vi "MotorRefNum_Simulation_Global.vi"(0 "menu":enum16{"set", "get", "delete"}(ring)=enum."get", 7 "PWM Channel":T1=enum."PWM 1", 9 "DC Motor Controller Set":refnum<class "DC Motor Controller.lvclass">, 11 "error in (no error)":errorcluster) -> (10 "DC Motor Controller Get":refnum<class "DC Motor Controller.lvclass">, 15 "error out":errorcluster)   [LabVIEW 2017]
doc: "Sets a reference into a registry, gets a reference from a registry, or deletes a reference from a registry. The reference is accessed by name, and can be given any unique name.\n\nThis software is licensed. Open the labview\\readme\\WPI Robotics Library Open Source License.txt file for more information."
uses:
  <instrlib>/DC Motor Controller/HAIOL/DC Motor Controller.lvclass
  <vilib>/Rock Robotics/SystemInterfaces/DIO/FPGA_DIOPWMChannel.ctl
panel:
  out "Array":refnum<class "DC Motor Controller.lvclass">[](array[class])
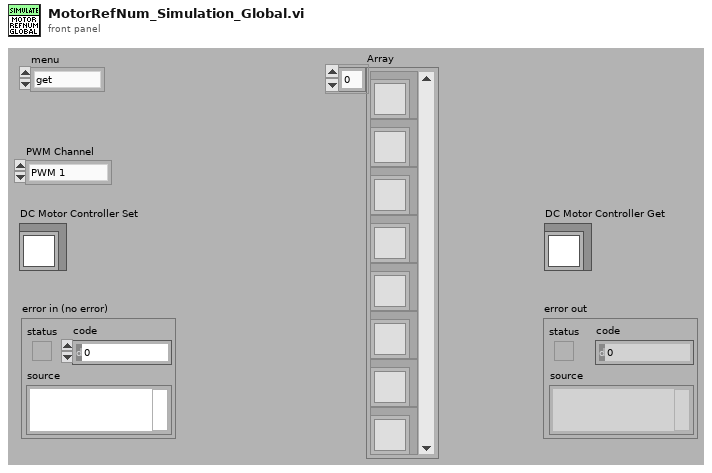
[diagram p1: front panel]
types:
  T1 = typedef "FPGA_DIOPWMChannel.ctl" = enum8{"PWM 0", "PWM 1", "PWM 2", "PWM 3", "PWM 4", "PWM 5", "PWM 6", "PWM 7", "PWM 8", "PWM 9", "PWM MXP 0", "PWM MXP 1", "PWM MXP 2", "PWM MXP 3", "PWM MXP 4", "PWM MXP 5", "PWM MXP 6", "PWM MXP 7", "PWM MXP 8", "PWM MXP 9", "Invalid"}
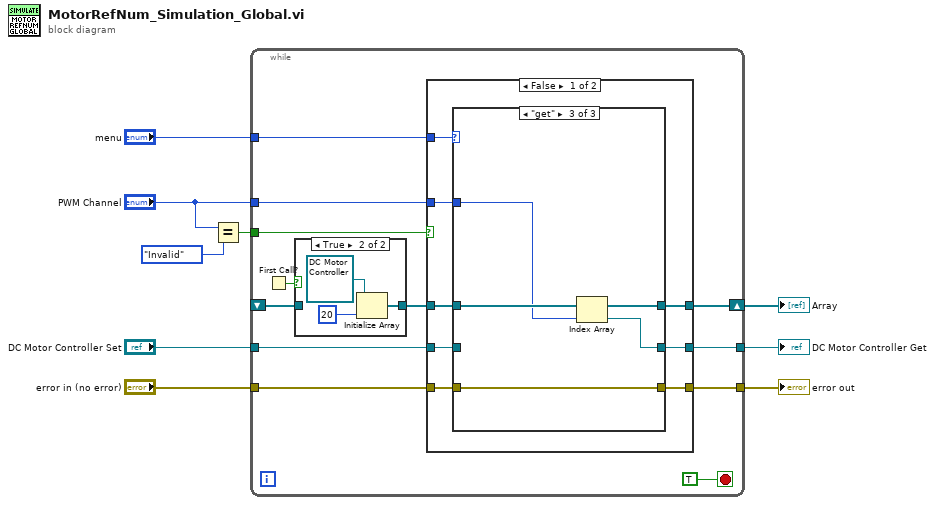
[diagram p0: block diagram]
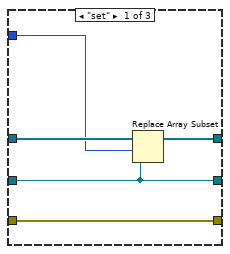
[diagram p2: hidden frame]
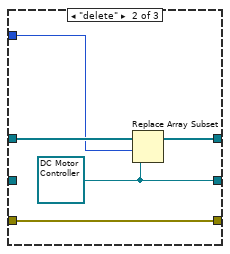
[diagram p3: hidden frame]
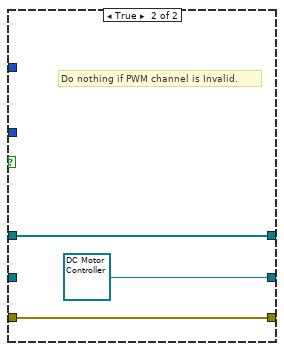
[diagram p4: hidden frame]
diagram:
  n1 = Equal?(x="PWM Channel", y=FPGA_DIOPWMChannel."Invalid" ("PWM Channel")) -> (x = y?=w6:bool)
  n2 = while {
    tunnel: "DC Motor Controller Set" -> [w21]
    tunnel: "error in (no error)" -> [w17]
    shift-right: [w20] -> w3
    shift-left: _ -> [w12]
    tunnel: [w19] -> w4
    tunnel: "menu" -> [w18]
    tunnel: [w16] -> w8
    tunnel: "PWM Channel" -> [w11]
    tunnel: w6 -> [w10]
    stop <- TRUE stop-if-true
    n3 = First Call?() -> (First Call?: T/F=w14:bool)
    n4 = case shown="True" w14 {
      tunnel: [w47 w49] -> w13
      tunnel: w12 -> [w47 _]
      frame False {
      }
      frame True {
        n5 = Initialize Array(refnum<class "DC Motor Controller.lvclass"> refnum ("DC Motor Controller Set"), 20 ("dimension size")) -> (w49:refnum<class "DC Motor Controller.lvclass">[])
      }
    }
    n6 = case shown="False" w10 {
      tunnel: w21 -> [w29 _]
      tunnel: [w28 w46] -> w20
      tunnel: [w27 refnum<class "DC Motor Controller.lvclass"> refnum ("DC Motor Controller Set")] -> w19
      tunnel: w18 -> [w26 _]
      tunnel: w17 -> [w25 w45]
      tunnel: [w24 w45] -> w16
      tunnel: w13 -> [w23 w46]
      tunnel: w11 -> [w22 _]
      frame False {
        n7 = case shown="\"get\"" w26 {
          tunnel: w29 -> [w32 _ _]
          tunnel: [w33 w38 w43] -> w28
          tunnel: w23 -> [w34 w39 w43]
          tunnel: [w32 w35 w42] -> w27
          tunnel: [w31 w37 w41] -> w24
          tunnel: w25 -> [w31 w37 w41]
          tunnel: w22 -> [w30 w36 w40]
          frame "set" {
            n8 = Replace Array Subset(array=w34, new element=w32, index=w30) -> (w33:refnum<class "DC Motor Controller.lvclass">[])
          }
          frame "delete" {
            w35 = refnum<class "DC Motor Controller.lvclass"> refnum ("DC Motor Controller Set")
            n9 = Replace Array Subset(array=w39, new element=w35, index=w36) -> (w38:refnum<class "DC Motor Controller.lvclass">[])
          }
          frame "get" {
            n10 = Index Array(array=w43, index=w40) -> (element=w42:refnum<class "DC Motor Controller.lvclass">)
          }
        }
      }
      frame True {
        # "Do nothing if PWM channel is Invalid."
      }
    }
  }
  "error out" <- w8
  "DC Motor Controller Get" <- w4
  "Array" <- w3
